vi "Prussure.vi"() -> ()   [LabVIEW 2015]
uses:
  <vilib>/Waveform/WDTOps.llb/WDT Append Waveforms DBL.vi
panel:
  out "Waveform Chart 2":waveform(dbl)(graph)
  out "Waveform Chart":waveform(dbl)(graph)
  in  "number of samples":i32=10
  in  "rate":dbl
  in  "stop":bool
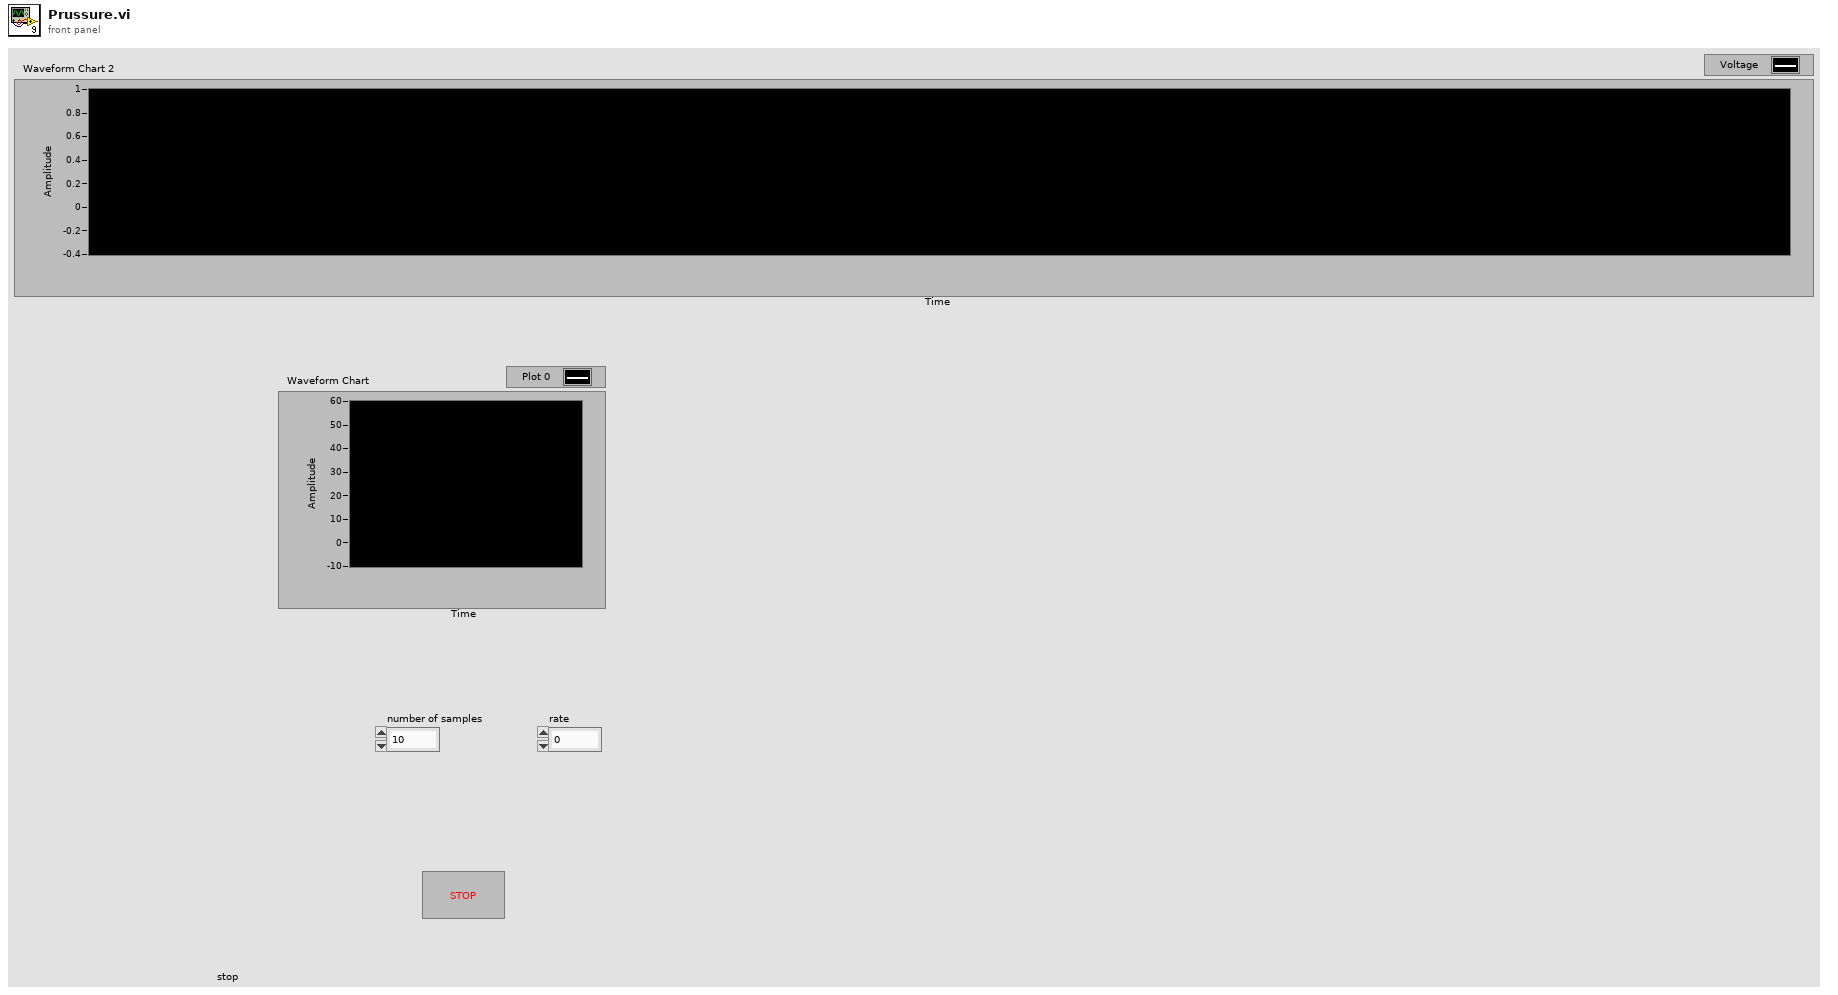
[diagram p1: front panel]
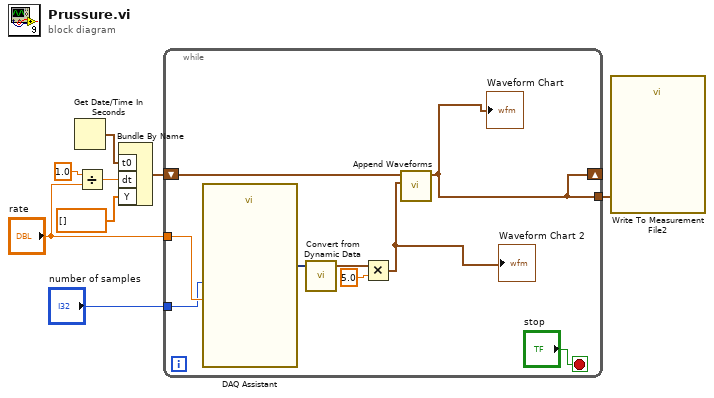
[diagram p0: block diagram]
diagram:
  n1 = Get Date/Time In Seconds() -> (seconds since 1Jan1904=w7:timestamp)
  n2 = Divide(x=1.0, y="rate") -> (x/y=w5:dbl)
  n3 = Bundle By Name("t0"=w7, "dt"=w5, "Y"=dbl[] []) -> (w8:waveform(dbl))  [unwired: 1 in]
  n4 = while {
    shift-right: [w10] -> _
    shift-left: w8 -> [w14]
    tunnel: "rate" -> [w16]
    tunnel: "number of samples" -> [w15]
    tunnel: [w10] -> w1
    stop <- "stop" stop-if-true
    n5 = call "DAQ Assistant"("rate"=w16, "number of samples"=w15) -> ("data"=w13:dynamicdata)  [unwired: 15 in, 2 out]
    n6 = call "Convert from Dynamic Data"("Dynamic Data Type"=w13) -> ("Waveform"=w12:waveform(dbl))  [unwired: 3 in]
    n7 = Multiply(x=w12, y=5.0) -> (x*y=w9:waveform(dbl))
    "Waveform Chart 2" <- w9
    n8 = call-poly <vilib>:"Append Waveforms.vi"("waveform B"=w9, "waveform A"=w14) -> ("waveform out"=w10:waveform(dbl))  [unwired: 8 in, 1 out]
    "Waveform Chart" <- w10
  }
  n9 = call "Write To Measurement File2"("Signals"=w1) -> ()  [unwired: 16 in, 3 out]
